vi "getTopics_Reply.vi"(7 "Code":i32, 8 "StatusMessage":string, 10 "Topic Types":string[](array[string]), 11 "Topics":string[](array[string])) -> (3 "XML Out":string="HTTP/1.1 200 OK\r\nServer: BaseHTTP/Labview\nDate: Wed, 23 Apr 2014 09:22:32 EST\r\nContent-Type: text/xml\r\nContent-Length: 511\r\n\r\n<?xml version='1.0'?>\n<methodResponse>\r <params>\r  <array>\r   <data>\r    <value>\r       <array>\r          <data>\r             <value><string>topic2</string> </value>\r             <value><string>type1</string> </value>\r          </data>\r       </array>\r    </value>\r    <value>\r       <array>\r          <data>\r             <value><string>topic2</string> </value>\r             <value><string>type2</string> </value>\r          </data>\r       </array>\r    </value>\r   </data>\r  </array>\r </params>\r</methodResponse>")   [LabVIEW 2012]
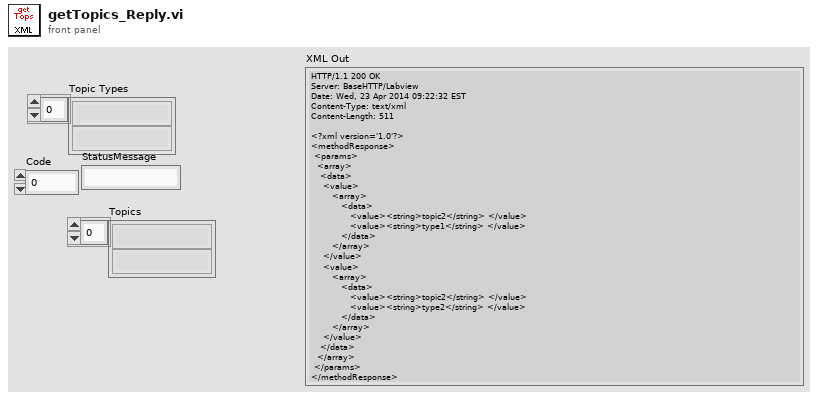
[diagram p1: front panel]
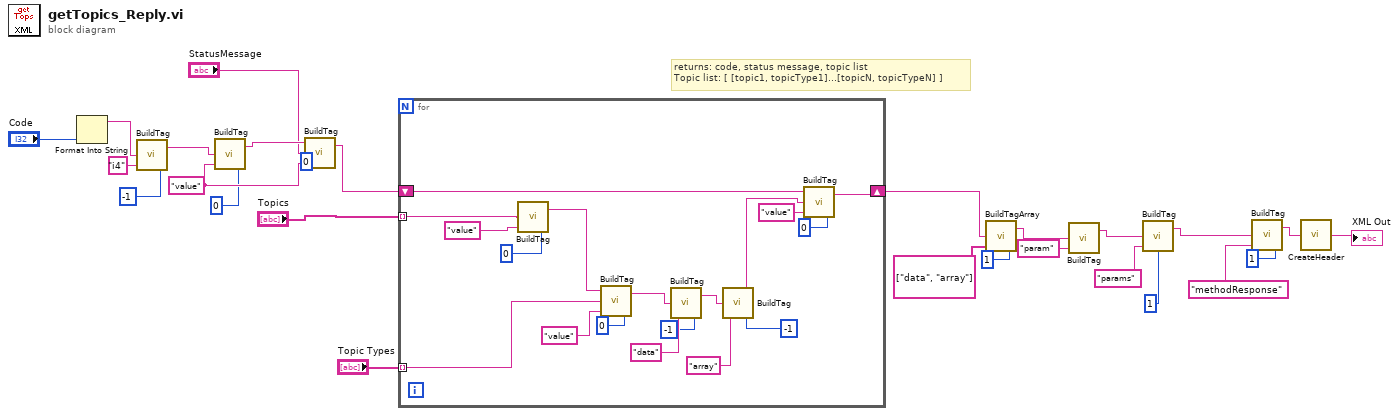
[diagram p0: block diagram]
diagram:
  w5 = "value" ("tag")
  # "returns: code, status message, topic list\nTopic list: [ [topic1, topicType1]...[topicN, topicTypeN] ]"
  n1 = Format Into String("Code") -> (resulting string=w9:string)  [unwired: 3 in, 1 out]
  n2 = call "BuildTag.vi"("Indent"=i8 -1, "tag"="i4", "value"=w9) -> ("string out"=w8:string)  [unwired: 1 in]
  n3 = call "BuildTag.vi"("Indent"=i8 0, "tag"=w5, "value"=w8) -> ("string out"=w7:string)  [unwired: 1 in]
  n4 = call "BuildTag.vi"("Indent"=i8 0, "tag"=w5, "value"="StatusMessage", "string in"=w7) -> ("string out"=w4:string)
  n5 = for {
    tunnel: "Topics" -> [w40] mode=indexing
    tunnel: "Topic Types" -> [w39] mode=indexing
    shift-right: [w38] -> w23
    shift-left: w4 -> [w37]
    n6 = call "BuildTag.vi"("Indent"=i8 0, "tag"="value", "value"=w40) -> ("string out"=w41:string)  [unwired: 1 in]
    n7 = call "BuildTag.vi"("Indent"=i8 0, "tag"="value", "value"=w39, "string in"=w41) -> ("string out"=w34:string)
    n8 = call "BuildTag.vi"("Indent"=i8 -1, "tag"="data", "value"=w34) -> ("string out"=w31:string)  [unwired: 1 in]
    n9 = call "BuildTag.vi"("Indent"=i8 -1, "tag"="array", "value"=w31) -> ("string out"=w30:string)  [unwired: 1 in]
    n10 = call "BuildTag.vi"("Indent"=i8 0, "tag"="value", "value"=w30, "string in"=w37) -> ("string out"=w38:string)
  }
  n11 = call "BuildTagArray.vi"("Indent"=i8 1, "tags"=string[] ["data", "array"], "value"=w23) -> ("string out"=w14:string)  [unwired: 1 in]
  n12 = call "BuildTag.vi"("tag"="param", "value"=w14) -> ("string out"=w12:string)  [unwired: 2 in]
  n13 = call "BuildTag.vi"("Indent"=i8 1, "tag"="params", "value"=w12) -> ("string out"=w18:string)  [unwired: 1 in]
  n14 = call "BuildTag.vi"("Indent"=i8 1, "tag"="methodResponse", "value"=w18) -> ("string out"=w21:string)  [unwired: 1 in]
  n15 = call "CreateHeader.vi"("Content"=w21) -> ("XML"=→"XML Out":string)
